vi "termometr_przelicznik.vi"() -> ()   [LabVIEW 2022 SP3]
panel:
  out "Stopnie":string
  in  "stop":bool
  out "?":dbl(knob) scale=35.0..120.0
  in  "C lub F":bool
  in  "Numeric":i16
  out "uwaga!!!":bool
  out "uwaga":bool
  in  "Knob":dbl(knob) scale=35.0..44.0
  out "Thermometer":dbl(slide) scale=35.0..44.0
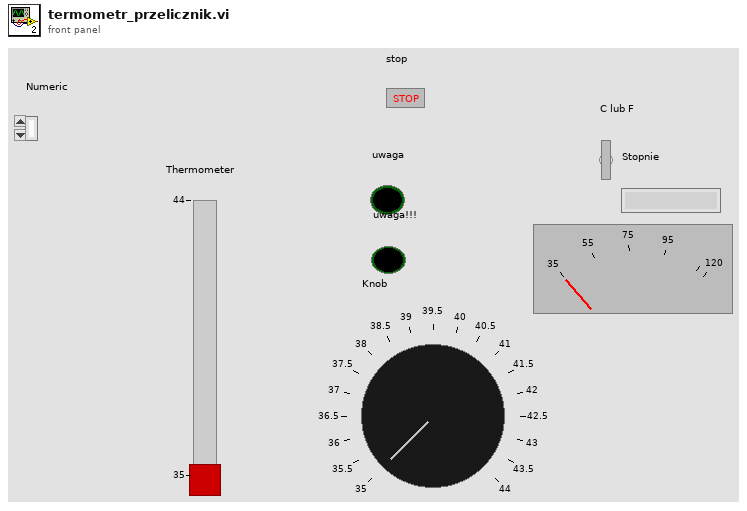
[diagram p1: front panel]
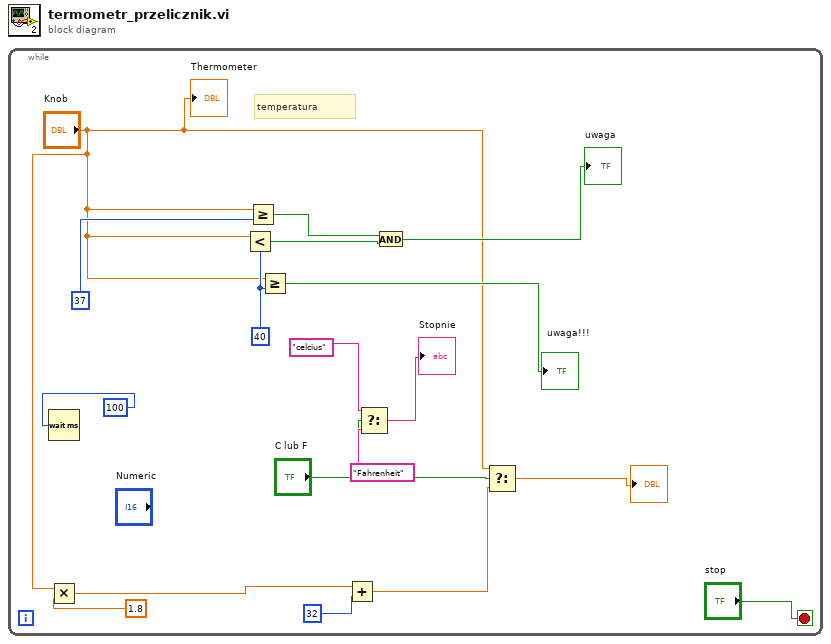
[diagram p0: block diagram]
diagram:
  n1 = while {
    stop <- "stop" stop-if-true
    w15 = 40
    # "temperatura"
    n2 = Wait (ms)(milliseconds to wait=u32 100) -> ()  [unwired: 1 out]
    n3 = Multiply(x="Knob", y=1.8) -> (x*y=w7:dbl)
    n4 = Less?(x="Knob", y=w15) -> (x < y?=w14:bool)
    n5 = Greater Or Equal?(x="Knob", y=37) -> (x >= y?=w16:bool)
    n6 = Greater Or Equal?(x="Knob", y=w15) -> (x >= y?=→"uwaga!!!":bool)
    n7 = Add(x=w7, y=32) -> (x+y=w5:dbl)
    n8 = Select(t="celcius" ("String"), s="C lub F", f="Fahrenheit" ("String")) -> (s? t:f=→"Stopnie":string)
    n9 = And(x=w16, y=w14) -> (x .and. y?=→"uwaga":bool)
    n10 = Select(t="Knob", s="C lub F", f=w5) -> (s? t:f=→"?":dbl)
    "Thermometer" <- "Knob"
  }
